vi "Global User_Answer.vi"() -> ()   [LabVIEW 2020]
panel:
  out "Answer":dbl
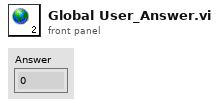
[diagram p1: front panel]
diagram:
